vi "AddPosition.vi"(8 "error in (no error)":errorcluster, 11 "Snake in":refnum<class "SnakeGame.lvclass">) -> (0 "error out":errorcluster, 3 "Snake out":refnum<class "SnakeGame.lvclass">)   [LabVIEW 2019, in "RT_Game.lvlib" / "SnakeGame.lvclass"]
uses:
  SnakeGame.lvclass
  SnakeGame.lvclass/SnakeGame.ctl
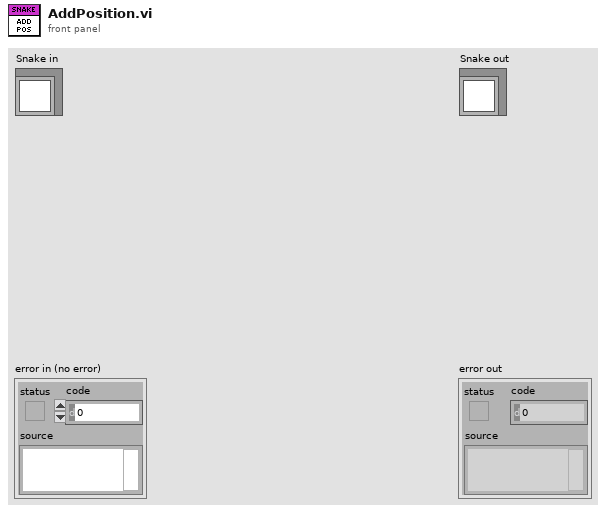
[diagram p1: front panel]
types:
  T1 = typedef "RT_Game.lvlib/SnakeGame.lvclass/SnakeData.ctl" = cluster{"Length":i16, "Direction":T2, "Position":T3, "Coordinates":T4[], "ScorePosition":T3, "Dead?":bool, "Color":fxp<+,3,3>, "LastDirection":T2}
  T2 = typedef "RT_Game.lvlib/SnakeGame.lvclass/Direction.ctl" = enum16{"Up", "Left", "Down", "Right"}
  T3 = typedef "RT_Game.lvlib/Game.lvclass/Coordinate.ctl" = cluster{"x":dbl, "y":dbl}
  T4 = typedef "RT_Game.lvlib/SnakeGame.lvclass/CoordinateData.ctl" = cluster{"Coordinate":T3, "TileCode":u16}
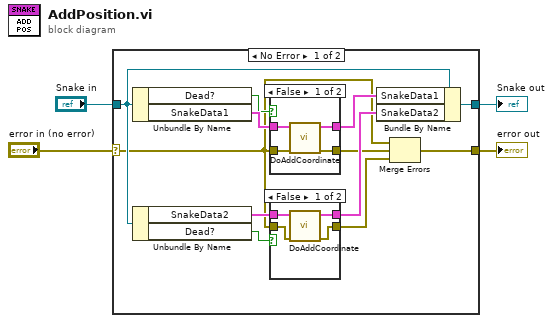
[diagram p0: block diagram]
diagram:
  n1 = case shown="No Error" "error in (no error)" {
    selector: "error in (no error)" -> [w8 w30]
    tunnel: [w7 w30] -> w3
    tunnel: [w16 w29] -> w1
    tunnel: "Snake in" -> [w14 w29]
    frame No Error {
      n2 = Unbundle By Name(w14) -> ("Dead?"=w13:bool, "SnakeData1"=w15:T1)
      n3 = Unbundle By Name(w14) -> ("SnakeData2"=w12:T1, "Dead?"=w11:bool)
      n4 = case shown="False" w13 {
        tunnel: [w20 w22] -> w10
        tunnel: w15 -> [w19 w22]
        tunnel: w8 -> [w18 w21]
        tunnel: [w17 w21] -> w6
        frame False {
          n5 = call "DoAddCoordinate.vi"("error in (no error)"=w18, "SnakeData1"=w19) -> ("error out"=w17:errorcluster, "SnakeData1 2"=w20:T1)  [unwired: 8 in]
        }
        frame True {
        }
      }
      n6 = case shown="False" w11 {
        tunnel: w12 -> [w26 w28]
        tunnel: [w25 w28] -> w9
        tunnel: w8 -> [w24 w27]
        tunnel: [w23 w27] -> w5
        frame False {
          n7 = call "DoAddCoordinate.vi"("error in (no error)"=w24, "SnakeData1"=w26) -> ("error out"=w23:errorcluster, "SnakeData1 2"=w25:T1)  [unwired: 8 in]
        }
        frame True {
        }
      }
      n8 = Bundle By Name(cluster=w14, "SnakeData1"=w10, "SnakeData2"=w9) -> (w16:refnum<class "SnakeGame.lvclass">)
      n9 = Merge Errors(w8, w6, w5) -> (w7:errorcluster)
    }
    frame Error {
    }
  }
  "error out" <- w3
  "Snake out" <- w1
